vi "LvMPDC_CMD_listallinfo.vi"(6 "timeout_ms":i32=25000, 8 "error in (no error)":errorcluster, 9 "ReadBytes":i32=1024, 10 "filepath":path, 11 "Connect ID":refnum<k5>) -> (0 "error out":errorcluster, 1 "playlist path[]":path[](array[path]), 3 "Connect ID out":refnum<k5>)   [LabVIEW 2012]
panel:
  # "LvMPDC:: CMD listallinfo"
  # "file: musiclibrary/BlueOysterCult/BurninForYou.mp3\nLast-Modified: 2015-02-07T00:09:56Z\nTime: 272\nArtist: Blue Oyster Cult\nAlbumArtist: Blue Oyster Cult\nTitle: Burnin' for You\nAlbum: Fire of Unknown Origin\nTrack: 2\nDate: 1981\nGenre: Other\nComposer: Donald Roeser/Richard Meltzer"
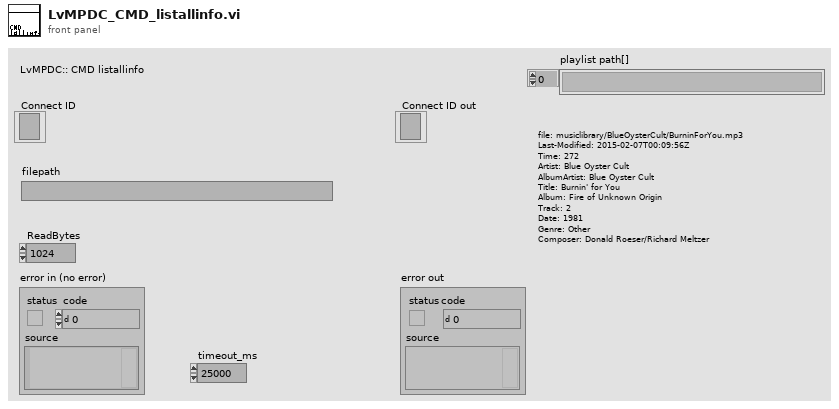
[diagram p1: front panel]
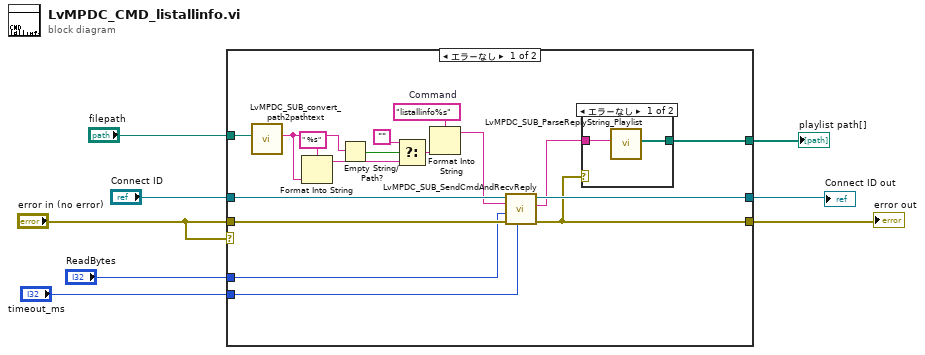
[diagram p0: block diagram]
diagram:
  n1 = case shown="エラーなし" "error in (no error)" {
    tunnel: "Connect ID" -> [w24 w29]
    tunnel: "error in (no error)" -> [w25 w28]
    tunnel: [w23 w29] -> w7
    tunnel: [w20 w28] -> w6
    tunnel: "timeout_ms" -> [w21 _]
    tunnel: "ReadBytes" -> [w22 _]
    tunnel: [w18 _] -> w2
    tunnel: "filepath" -> [w17 _]
    frame No Error {
      w9 = "listallinfo%s"  # Command
      n2 = call "LvMPDC_SUB_convert_path2pathtext.vi"("path"=w17) -> ("pathtext"=w13:string)  [unwired: 10 in]
      n3 = Format Into String(format string=" %s" ("形式文字列"), w13) -> (resulting string=w10:string)  [unwired: 2 in, 1 out]
      n4 = Empty String/Path?(string/path=w13) -> (empty?=w12:bool)
      n5 = Select(t="", s=w12, f=w10) -> (s? t:f=w14:string)
      n6 = Format Into String(format string=w9, w14) -> (resulting string=w16:string)  [unwired: 2 in, 1 out]
      n7 = call "LvMPDC_SUB_SendCmdAndRecvReply.vi"("timeout_ms"=w21, "error in (no error)"=w25, "ReadBytes"=w22, "Command"=w16, "Connect ID"=w24) -> ("error out"=w20:errorcluster, "Reply"=w19:string, "Connect ID out"=w23:refnum<k5>)  [unwired: 4 in]
      n8 = case shown="エラーなし" w20 {
        tunnel: w19 -> [w27 _]
        tunnel: [w26 _] -> w18
        frame No Error {
          n9 = call "LvMPDC_SUB_ParseReplyString_Playlist.vi"("string"=w27) -> ("playlist path[]"=w26:path[])  [unwired: 10 in]
        }
        frame Error {
        }
      }
    }
    frame Error {
    }
  }
  "Connect ID out" <- w7
  "error out" <- w6
  "playlist path[]" <- w2
